vi "ncs_v3.vi"() -> ()   [LabVIEW 2016]
uses:
  <instrlib>/niUSRP/niUSRP Timestamp.ctl
  <instrlib>/niUSRP/niUSRP Write Tx Data (2D CDB).vi
  <instrlib>/niUSRP/niUSRP Fetch Rx Data (2D CDB).vi
panel:
  out "Coerced Rx IQ Rate":dbl
  in  "Sampling Rate":i32=500
  out "Gain":dbl=-15.0
  out "Bandwidth":dbl=56000000.0
  out "Coerced Carrier Frequency":dbl=2000000000.0 format="%#.17g"
  out "Coerced Tx IQ rate":dbl=1000000.0
  out "error IO":errorcluster={"status"=FALSE, "code"=-1074118647, "source"=""}
  in  "Rx Number of Samples":i32=20000
  in  "Tab Control 2":enum32{"NI-294x/295x", "NI-2900/2901"}(tab)=enum."NI-2900/2901"
  in  "Rx carrier frequency [Hz]":dbl=2000000000.0 format="%#_6p"
  in  "Tx carrier frequency [Hz]":dbl=1000000000.0 format="%#_6p"
  in  "Start Trigger Time":T1={"whole seconds"=1, "fractional seconds"=0.0}
  in  "Tab Control":T2(tab)
  out "NCS tag Amp":dbl[](graph)=[0.011967714738528729, 0.012021355192189592, 0.012015275039596582, 0.011969166030167903, 0.011958890166168242, 0.012007893820858737, 0.012022893722444085, 0.011978222225113794, 0.011969989939463181, 0.012003099640895068]
  out "NCS tag Phase":dbl[](graph)=[0.011967714738528729, 0.012021355192189592, 0.012015275039596582, 0.011969166030167903, 0.011958890166168242, 0.012007893820858737, 0.012022893722444085, 0.011978222225113794, 0.011969989939463181, 0.012003099640895068]
  out "Tag Amp":dbl[](graph)
  out "Tag Phase":dbl[](graph)
  out "Tx Waveform Graph":waveform(dbl)[](graph)
  in  "Stop":bool
  in  "Channel 0\nTone Amplitude":dbl=0.707 step=0.05 format="%#.6g"
  in  "Channel 0 \nTone Frequency":dbl=5000.0 format="%#_6p"
  in  "Tx Waveform Size":dbl=2000.0
  in  "Device Name":refnum<k15>="MyB210"
  in  "Tx Gain":dbl=28.0 format="%#_6f"
  in  "Tx IQ Rate":dbl=1000000.0 format="%#_6p"
  in  "Rx Gain":dbl=32.0 format="%#_6f"
  in  "Rx IQ Rate":dbl=1000000.0 format="%#_6p"
  # "Rx Settings"
  # "Tx Settings"
  # "Note that on the NI-2900 and NI-2901, both Rx channels share an LO and both Tx channels share an LO. However, on the NI-294x/295x devices, Rx and Tx of channel 0 share an LO and Rx and Tx of channel 1 share an LO."
  # "This Tx graph should always have end and start tied up since this is being sent in a loop continuously. Otherwise phase jumps will be noticed."
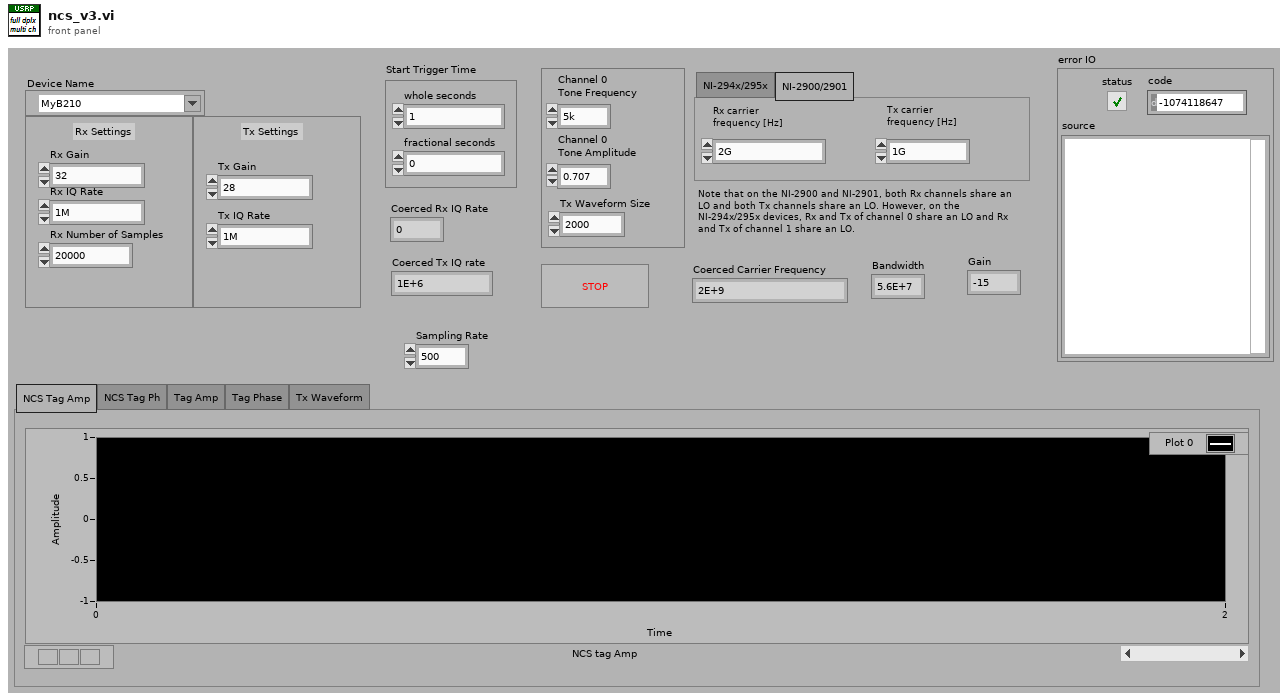
[diagram p1: front panel]
types:
  T1 = typedef "niUSRP Timestamp.ctl" = cluster{"whole seconds":u64, "fractional seconds":dbl}
  T2 = enum32{"NCS Tag Amp", "NCS Tag Ph", "Tag Amp", "Tag Phase", "Tx Waveform"}
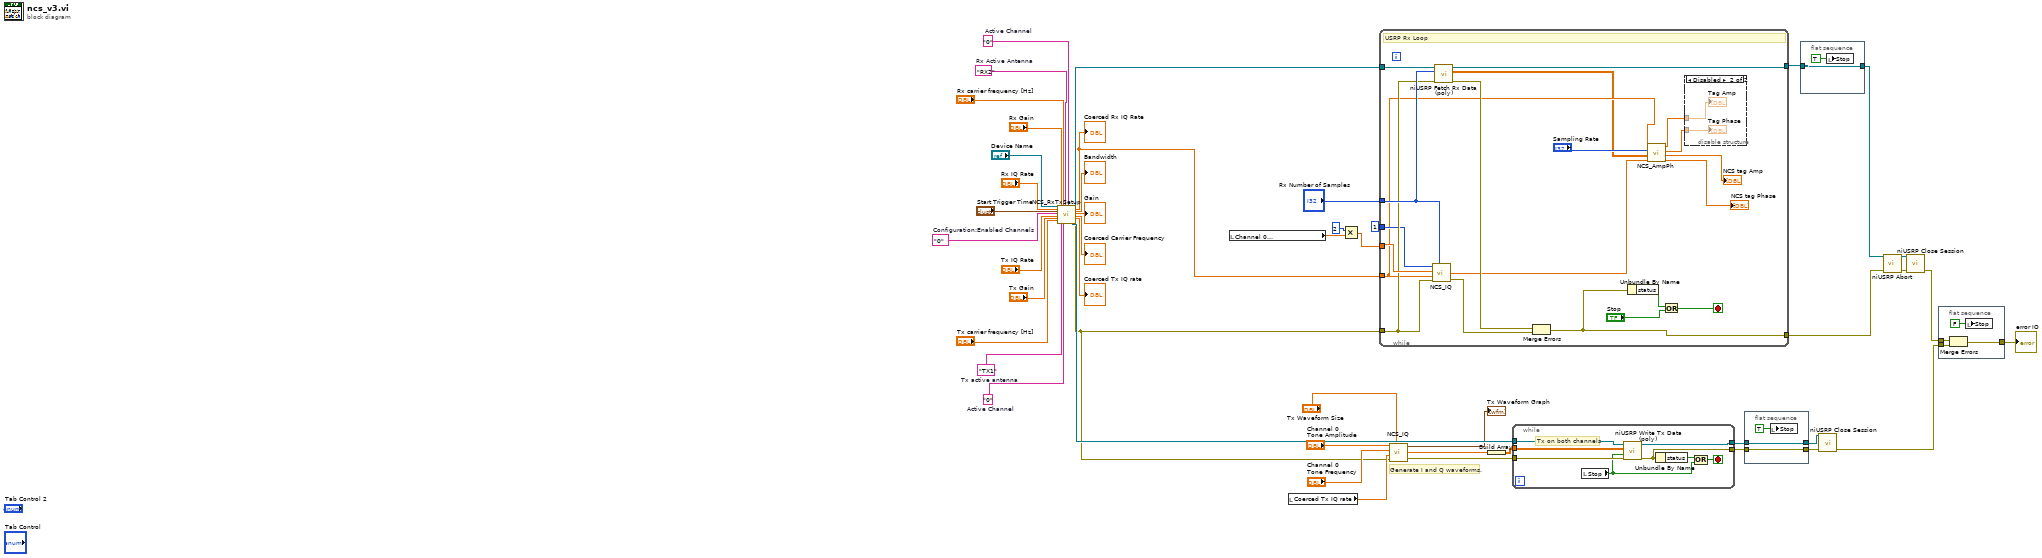
[diagram p0: block diagram]
diagram:
  w2 = "0"  # Active Channel
  w3 = "0"  # Active Channel
  w38 = "RX2"  # Rx Active Antenna
  w34 = "TX1"  # Tx active antenna
  w20 = "0"  # Configuration:Enabled Channels
  # "Generate I and Q waveforms."
  n1 = call "NCS_RxTxSetup.vi"("IVI Refnum in"="Device Name", "Rx IQ Rate"="Rx IQ Rate", "Start Trigger Time"="Start Trigger Time", "Configuration:Enabled Channels"=w20, "Tx IQ Rate"="Tx IQ Rate", "Tx Gain"="Tx Gain", "Tx carrier frequency [Hz]"="Tx carrier frequency [Hz]", "Rx Gain"="Rx Gain", "Tx active antenna"=w34, "Rx carrier frequency [Hz]"="Rx carrier frequency [Hz]", "Active Channel"=w2, "Rx Active Antenna"=w38, "Active Channel 2"=w3) -> ("session handle out"=w45:refnum<k15>, "IVI Refnum out"=w46:refnum<k15>, "Coerced Rx IQ Rate"=w1:dbl, "Bandwidth"=→"Bandwidth":dbl, "Gain"=→"Gain":dbl, "Carrier Frequency"=→"Coerced Carrier Frequency":dbl, "IQ Rate 2"=→"Coerced Tx IQ rate":dbl, "error out"=w13:errorcluster)  [unwired: 7 in]
  "Coerced Rx IQ Rate" <- w1
  n2 = local read "Channel 0 \nTone Frequency"() -> (w19:dbl)
  n3 = local read "Coerced Tx IQ rate"() -> (w14:dbl)
  n4 = Multiply(x=2, y=w19) -> (x*y=w18:dbl)
  n5 = while {
    tunnel: w46 -> [w66]
    tunnel: w13 -> [w58]
    tunnel: [w65] -> w30
    tunnel: "Rx Number of Samples" -> [w60]
    tunnel: w1 -> [w54]
    tunnel: [w55] -> w22
    tunnel: w18 -> [w59]
    tunnel: 1 -> [w56]
    stop <- w61 stop-if-true
    # "USRP Rx Loop"
    n6 = call "NCS_IQ.vi"("Tone Amplitude"=w56, "Waveform Size"=w60, "Tone Frequency"=w59, "Coerced IQ rate"=w54, "error in (no error)"=w58) -> ("IQ waveform array"=w51:cdb[], "error out"=w57:errorcluster)  [unwired: 1 in, 1 out]
    n7 = call-poly <instrlib>:"niUSRP Fetch Rx Data (poly).vi"("session handle"=w66, "number of samples"=w60, "error in (no error)"=w58) -> ("session handle out"=w65:refnum<k15>, "data"=w52:cdb[][], "error out"=w62:errorcluster)  [unwired: 9 in, 1 out]
    n8 = Merge Errors(w62, w57) -> (w55:errorcluster)
    n9 = Unbundle By Name(w55) -> ("status"=w64:bool)
    n10 = call "NCS_AmpPh.vi"("IQ"=w51, "data"=w52, "Sampling Rate"="Sampling Rate", "Coerced Rx IQ Rate"=w54) -> ("Phase DownSampled"=→"NCS tag Phase":dbl[], "Amp DownSampled"=→"NCS tag Amp":dbl[], "Unfiltered Phase"=w49:dbl[], "Unfiltered Amplitude"=w50:dbl[])  [unwired: 4 in]
    n11 = Or(x=w64, y="Stop") -> (x .or. y?=w61:bool)
    n12 = disable-structure shown="Disabled" {
      disable-tunnel: w50 -> [_ w68]
      disable-tunnel: w49 -> [_ w67]
      frame Enabled {
      }
      frame Disabled {
        "Tag Amp" <- w68
        "Tag Phase" <- w67
      }
    }
  }
  n13 = call "NCS_IQ.vi"("Tone Amplitude"="Channel 0\nTone Amplitude", "Waveform Size"="Tx Waveform Size", "Tone Frequency"="Channel 0 \nTone Frequency", "Coerced IQ rate"=w14, "error in (no error)"=w13) -> ("IQ waveform"=→"Tx Waveform Graph":waveform(dbl)[], "IQ waveform array"=w11:cdb[], "error out"=w12:errorcluster)  [unwired: 1 in]
  n14 = Build Array(w11) -> (w42:cdb[][])
  n15 = while {
    tunnel: w45 -> [w76]
    tunnel: w12 -> [w75]
    tunnel: [w73] -> w33
    tunnel: [w71] -> w28
    tunnel: w42 -> [w69]
    stop <- w72 stop-if-true
    # "Tx on both channels"
    n16 = local read "Stop"() -> (w70:bool)
    n17 = call-poly <instrlib>:"niUSRP Write Tx Data (poly).vi"("session handle"=w76, "data"=w69, "end of data?"=w70, "error in (no error)"=w75) -> ("session handle out"=w71:refnum<k15>, "error out"=w73:errorcluster)  [unwired: 10 in]
    n18 = Unbundle By Name(w73) -> ("status"=w74:bool)
    n19 = Compound Arithmetic op=OR(w74, w70) -> (w72:bool)
  }
  n20 = flat-sequence {
    tunnel: [w78] -> w32
    tunnel: w33 -> [w78]
    tunnel: [w77] -> w29
    tunnel: w28 -> [w77]
    frame #0 {
      n21 = local write "Stop"(TRUE ("STOP")) -> ()
    }
  }
  n22 = flat-sequence {
    tunnel: [w80] -> w31
    tunnel: w30 -> [w80]
    frame #0 {
      n23 = local write "Stop"(TRUE ("STOP")) -> ()
    }
  }
  n24 = call <instrlib>:"niUSRP Close Session.vi"("session handle"=w29, "error in (no error)"=w32) -> ("error out"=w27:errorcluster)  [unwired: 13 in]
  n25 = call <instrlib>:"niUSRP Abort.vi"("session handle"=w31, "error in (no error)"=w22) -> ("session handle out"=w44:refnum<k15>, "error out"=w43:errorcluster)  [unwired: 12 in]
  n26 = call <instrlib>:"niUSRP Close Session.vi"("session handle"=w44, "error in (no error)"=w43) -> ("error out"=w24:errorcluster)  [unwired: 13 in]
  n27 = flat-sequence {
    tunnel: w27 -> [w84]
    tunnel: [w83] -> w25
    tunnel: w24 -> [w82]
    frame #0 {
      n28 = Merge Errors(w82, w84) -> (w83:errorcluster)
      n29 = local write "Stop"(FALSE ("STOP")) -> ()
    }
  }
  "error IO" <- w25
